vi "Semstatusvi.vi"() -> ()   [LabVIEW 2011]
panel:
  out "size":i32
  out "# waiting":i32
  out "# available":i32
  out "name":string
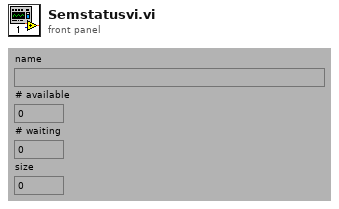
[diagram p1: front panel]
types:
  T1 = typedef "Semaphore RefNum" = refnum<k1>
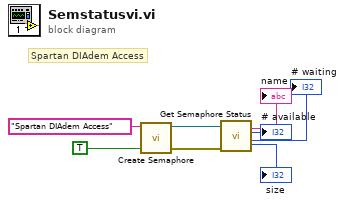
[diagram p0: block diagram]
diagram:
  # "Spartan DIAdem Access"
  n1 = call <vilib>:"Create Semaphore.vi"("return existing (F)"=TRUE, "name (unnamed)"="Spartan DIAdem Access") -> ("error out"=w5:errorcluster, "semaphore"=w6:T1)  [unwired: 2 in, 2 out]
  n2 = call <vilib>:"Get Semaphore Status.vi"("error in (no error)"=w5, "semaphore"=w6) -> ("# waiting"=→"# waiting":i32, "# available"=→"# available":i32, "size"=→"size":i32, "name"=→"name":string)  [unwired: 6 out]
